vi "Multicolumn Listbox add new row data - Copy.vi"(8 "error in (no error)":errorcluster, 10 "String":string, 11 "Multicolumn Listbox In":refnum<vi>) -> (0 "error out":errorcluster, 3 "Multicolumn Listbox Out":refnum<vi>)   [LabVIEW 2021]
panel:
  in  "Multicolumn Listbox":i32(listbox)
  in  "s":bool
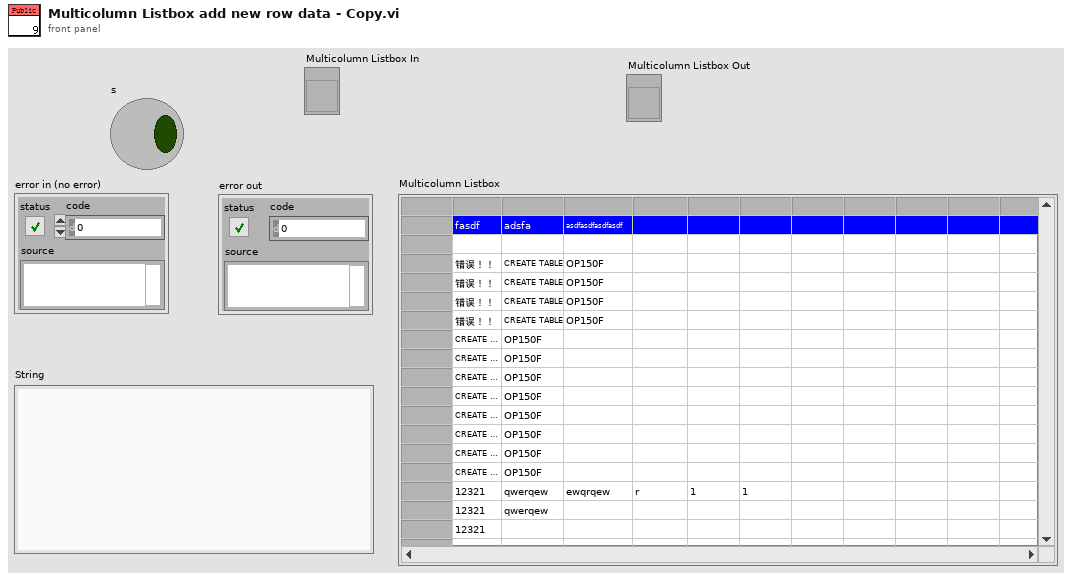
[diagram p1: front panel]
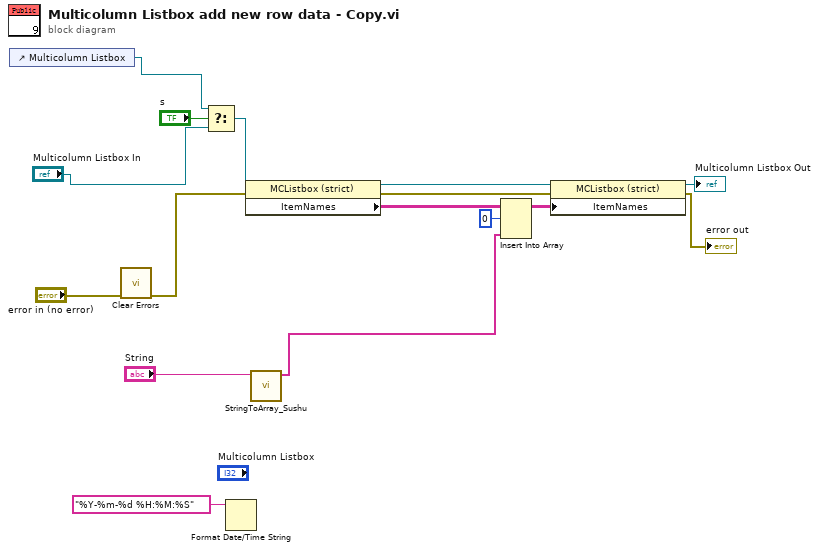
[diagram p0: block diagram]
diagram:
  n1 = control-ref of="Multicolumn Listbox"() -> (w8:refnum<vi>)
  n2 = call <vilib>:"Clear Errors.vi"("error in (no error)"="error in (no error)") -> ("error out"=w5:errorcluster)  [unwired: 5 in, 1 out]
  n3 = Select(t=w8, s="s", f="Multicolumn Listbox In") -> (s? t:f=w11:refnum<vi>)
  n4 = Format Date/Time String(time format string (%c)="%Y-%m-%d %H:%M:%S") -> ()  [unwired: 2 in, 1 out]
  n5 = property class="MCListbox (strict)"(reference=w11, error in=w5) -> (reference out=w14:refnum<vi>, error out=w13:errorcluster, "ItemNames"=w16:string[][])
  n6 = call <userlib>:"StringToArray_Sushu.vi"("State Queue"="String") -> ("Array"=w9:string[])  [unwired: 7 in, 3 out]
  n7 = Insert Into Array(array=w16, index (row)=0, new element=w9) -> (w15:string[][])  [unwired: 1 in]
  n8 = property class="MCListbox (strict)"(reference=w14, error in=w13, "ItemNames"=w15) -> (reference out=→"Multicolumn Listbox Out":refnum<vi>, error out=→"error out":errorcluster)
